vi "Get Picture.vi"(8 "error in (no error)":errorcluster, 11 "Device in":refnum<class "Device.lvclass">) -> (0 "error out":errorcluster, 2 "Device Pic":T1, 3 "Device out":refnum<class "Device.lvclass">)   [LabVIEW 2013, in "Device.lvclass"]
uses:
  Device.lvclass
  <vilib>/picture/picture.llb/imagedata.ctl
panel:
  in  "path to PNG file":path
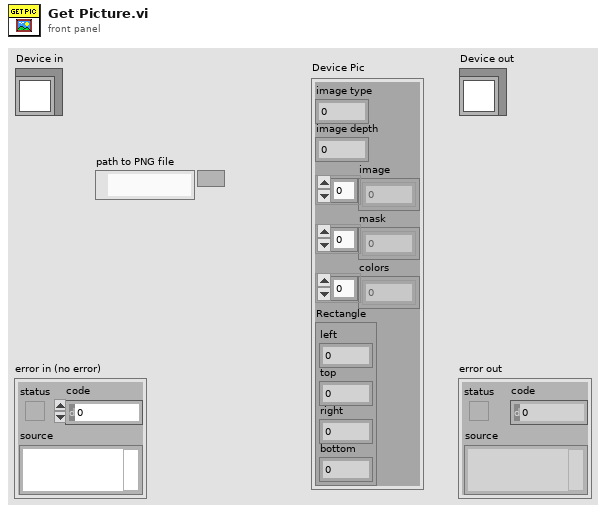
[diagram p1: front panel]
types:
  T1 = typedef "imagedata.ctl" = cluster{"image type":i32, "image depth":i32, "image":u8[], "mask":u8[], "colors":u32[], "Rectangle":cluster{"left":i16, "top":i16, "right":i16, "bottom":i16}}
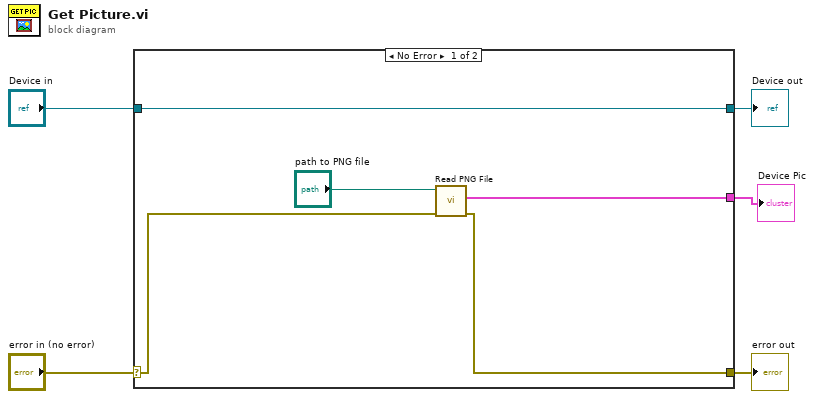
[diagram p0: block diagram]
diagram:
  n1 = case shown="No Error" "error in (no error)" {
    selector: "error in (no error)" -> [w9 w12]
    tunnel: [w8 w12] -> w4
    tunnel: [w10 w11] -> w2
    tunnel: "Device in" -> [w10 w11]
    tunnel: [w6 _] -> w1
    frame No Error {
      n2 = call <vilib>:"Read PNG File.vi"("error in (no error)"=w9, "path to PNG file"="path to PNG file") -> ("error out"=w8:errorcluster, "image data"=w6:T1)  [unwired: 7 in, 1 out]
    }
    frame Error {
    }
  }
  "error out" <- w4
  "Device out" <- w2
  "Device Pic" <- w1
